vi "Get - wForms.vi"(0 "reference in":refnum<class "GSwFormDSP.lvclass">, 5 "error in (no error)":errorcluster, 6 "Normalization Option":T1(ring), 7 "Indexes (Empty = ALL)":i32[](array[numeric])) -> (11 "Nb Signals":i32, 13 "wForms":waveform(dbl)[](array[waveform]), 14 "reference out":refnum<class "GSwFormDSP.lvclass">, 19 "error out":errorcluster)   [LabVIEW 2022 SP3, in "GSwFormDSP.lvclass"]
uses:
  GSwFormDSP.lvclass
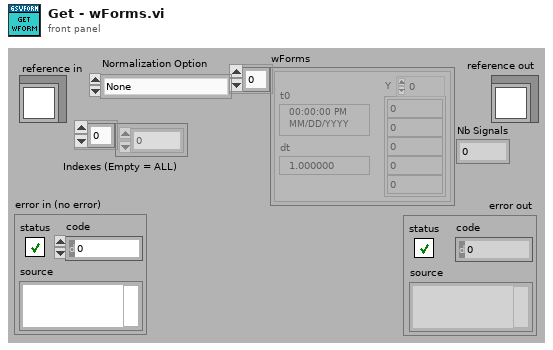
[diagram p1: front panel]
types:
  T1 = enum16{"None", "To itself", "To the max levels of ALL the signals"}
  T2 = typedef "GSwFormDSP.lvclass/ObjectAttributes.ctl" = cluster{"Wform Ref":refnum<data-value>, "Nb Signals":i32, "Spectral Function Parameters":T3, "FFT":waveform(cdb)[], "Nb FFT":i32, "Nb Averages":i32[], "Reference Indexes":i32[], "Response Indexes":i32[], "Coherence":waveform(dbl)[], "TDF Parameters":T5, "DAQ":cluster{"Duration (sec)":dbl, "Buffer Size (Samples)":i32, "Offset (Samples)":i32}, "Filter Impulse Response (TDF)":waveform(dbl), "Sound Playback":T6}
  T3 = typedef "GSwFormDSP.lvclass/Spectral Parameters.ctl" = cluster{"Frequency resolution (Hz)":dbl, "Overlap":dbl, "Window":T4}
  T4 = typedef "NI_AALPro.lvlib/windowTd.ctl" = u32
  T5 = typedef "GSwFormDSP.lvclass/TDF Parameters.ctl" = cluster{"Filter":enum32{"Lowpass", "Highpass", "Bandpass", "Bandstop"}, "Type:":enum16{"Butterworth", "Chebyshev", "Inv Chebyshev", "Elliptic", "Bessel"}, "LP cutoff freq":dbl, "HP cutoff freq":dbl, "Order":i32, "passband ripple (dB)":dbl, "stopband attenuation (dB)":dbl, "Phaseless Filter":bool, "Include Fade IN and OUT":bool}
  T6 = typedef "GSwFormDSP.lvclass/Sound Playback.ctl" = cluster{"Timer start (ms)":u32, "task ID":T7, "Cursor Init Location (s)":dbl, "SC Volume":dbl}
  T7 = typedef "Sound Output Task ID.ctl" = u32
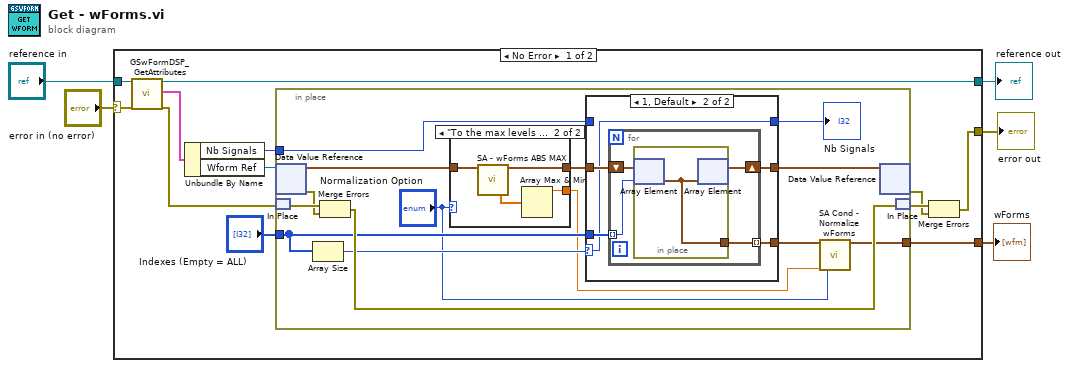
[diagram p0: block diagram]
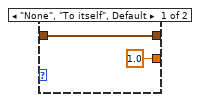
[diagram p2: hidden frame]
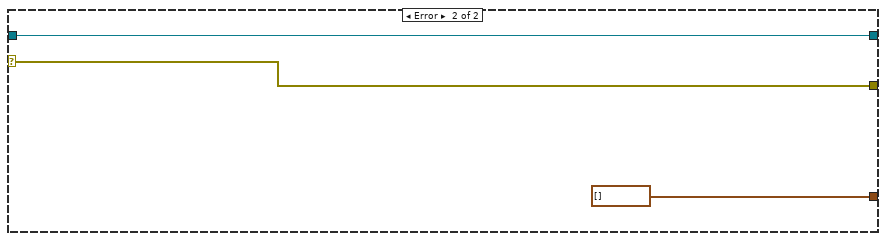
[diagram p4: hidden frame]
diagram:
  n1 = case shown="No Error" "error in (no error)" {
    selector: "error in (no error)" -> [w17 w52]
    tunnel: [w8 w52] -> w4
    tunnel: [w16 w51] -> w2
    tunnel: "reference in" -> [w15 w51]
    tunnel: [w7 waveform(dbl)[] []] -> w1
    frame No Error {
      n2 = call "GSwFormDSP_GetAttributes.vi"("reference in"=w15, "error in (no error)"=w17) -> ("reference out"=w16:refnum<class "GSwFormDSP.lvclass">, "attributes"=w14:T2, "error out"=w13:errorcluster)  [unwired: 14 in, 1 out]
      n3 = Unbundle By Name(w14) -> ("Nb Signals"=w6:i32, "Wform Ref"=w12:refnum<data-value>)
      n4 = in-place {
        in-place-border: "Indexes (Empty = ALL)" -> [w27]
        in-place-border: [w25] -> w7
        in-place-border: w6 -> [w22]
        n5 = in-place-dvr #1(w12) -> (w21:waveform(dbl)[], w29:errorcluster)
        n6 = in-place-match #2(w13) -> (w30:errorcluster)
        n7 = Array Size(array=w27) -> (size(s)=w26:i32)
        n8 = Merge Errors(w30, w29) -> (w31:errorcluster)
        n9 = case shown="\"To the max levels of ALL the signals\"" "Normalization Option" {
          tunnel: w21 -> [w33 w36]
          tunnel: [w33 w35] -> w20
          tunnel: [1.0 w34] -> w19
          frame "None", "To itself", Default {
          }
          frame "To the max levels of ALL the signals" {
            n10 = call "SA - wForms ABS MAX.vi"("wForms IN"=w36) -> ("ABS MAX's"=w37:dbl[], "wForms OUT"=w35:waveform(dbl)[])  [unwired: 17 in]
            n11 = Array Max & Min(array=w37) -> (max value=w34:dbl)  [unwired: 3 out]
          }
        }
        n12 = case shown="1, Default" w26 {
          selector: w26 -> [_ w40]
          tunnel: w20 -> [w39 w44]
          tunnel: w27 -> [_ w43]
          tunnel: [w39 w42] -> w28
          tunnel: [w39 w41] -> w24
          tunnel: [w38 w40] -> w23
          tunnel: w22 -> [w38 _]
          frame 0 {
          }
          frame 1, Default {
            n13 = for {
              shift-right: [w46] -> w42
              shift-left: w44 -> [w48]
              tunnel: w43 -> [w47] mode=indexing
              tunnel: [w45] -> w41 mode=indexing
              n14 = in-place {
                in-place-border: [w49] -> w45
                n15 = in-place-array #3(w48, w47) -> (w49:waveform(dbl))
                n16 = in-place-array #3(w49) -> (w46:waveform(dbl)[])  [unwired: 1 out]
              }
            }
          }
        }
        "Nb Signals" <- w23
        n17 = call "SA Cond - Normalize wForms.vi"("wForms IN"=w24, "Max of ALL Signals"=w19, "Normalization Option"="Normalization Option") -> ("wForms OUT"=w25:waveform(dbl)[])  [unwired: 16 in]
        n18 = in-place-dvr #1(w28) -> (w9:errorcluster)  [unwired: 1 out]
        n19 = in-place-match #2(w31) -> (w10:errorcluster)
      }
      n20 = Merge Errors(w10, w9) -> (w8:errorcluster)
    }
    frame Error {
    }
  }
  "error out" <- w4
  "reference out" <- w2
  "wForms" <- w1
